vi "Read Event Log Credentials.vi"(11 "IMediator in":refnum<class "IMediator.lvclass">) -> (1 "Framework Instance Alias":string, 2 "Event Log Instance":refnum<class "LoggerReference.lvclass">)   [LabVIEW 2018, in "MVA Framework.lvlib" / "IMediator.lvlib" / "IMediator.lvclass"]
doc: "读取事件日志凭据"
uses:
  IMediator.lvclass
  composed-event-logger/Source/Composed Log/LoggerReference/LoggerReference.lvclass
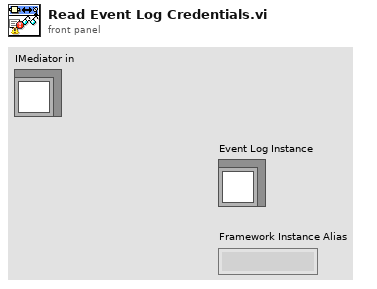
[diagram p1: front panel]
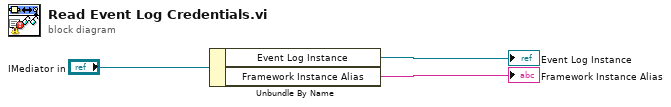
[diagram p0: block diagram]
diagram:
  n1 = Unbundle By Name("IMediator in") -> ("Event Log Instance"=→"Event Log Instance":refnum<class "LoggerReference.lvclass">, "Framework Instance Alias"=→"Framework Instance Alias":string)
